vi "QueueDequeue.vi"(8 "error in (no error)":errorcluster, 11 "Execute":refnum<class "Execute.lvclass">) -> (0 "error out":errorcluster, 1 "Stop":bool, 2 "Interface Message":refnum<class "Interface Message.lvclass">, 3 "Execute":refnum<class "Execute.lvclass">)   [LabVIEW 2018, in "QMH_Class.lvlib" / "TestManager.lvlib" / "Execute.lvclass"]
uses:
  Execute.lvclass
  Message_class/InterfaceMessage/Interface Message.lvclass
  Message_class/StopMessage/Stop Message.lvclass
  Execute.lvclass/Execute.ctl
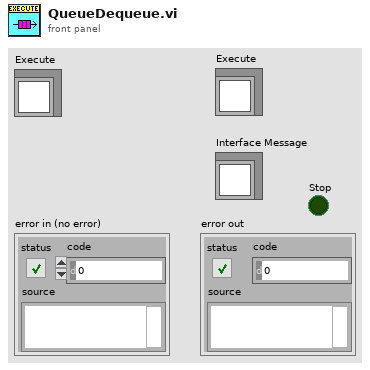
[diagram p1: front panel]
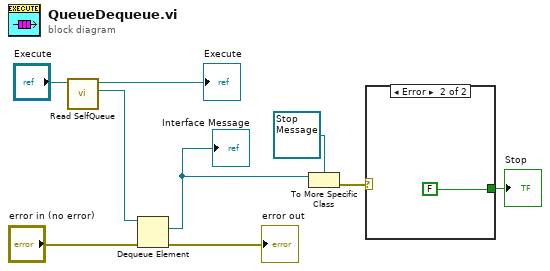
[diagram p0: block diagram]
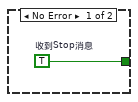
[diagram p2: hidden frame]
diagram:
  n1 = call "Read SelfQueue.vi"("Execute"="Execute") -> ("SelfQueue"=w8:refnum<queue>, "Execute"=→"Execute":refnum<class "Execute.lvclass">)  [unwired: 8 in, 1 out]
  n2 = Dequeue Element(queue=w8, error in (no error)="error in (no error)") -> (element=w4:refnum<class "Interface Message.lvclass">, error out=→"error out":errorcluster)  [unwired: 1 in, 2 out]
  "Interface Message" <- w4
  n3 = To More Specific Class(target class=refnum<class "Stop Message.lvclass"> refnum ("QMH_Class.lvlib:TestManager.lvlib:Stop Message.lvclass"), reference=w4) -> (error out=w2:errorcluster)  [unwired: 1 in, 1 out]
  n4 = case shown="Error" w2 {
    tunnel: [w10 FALSE] -> w1
    frame No Error {
      w10 = TRUE  # 收到Stop消息
    }
    frame Error {
    }
  }
  "Stop" <- w1
